vi "AprilTagFieldLayout_GetField.vi"(11 "AprilTagFieldLayout":T6={"AprilTagMap"={}, "FieldLength"=0.0, "FieldWidth"=0.0, "OriginPosition "=enum."kBlueAllianceWallRightSide,", "OriginPose3d"={"Translation3d"={"X"=0.0, "Y"=0.0, "Z"=0.0}, "Rotation3d"={"Q_quaternion"={"R"=1.0, "V"=[0.0, 0.0, 0.0]}}}} {"OriginPose3d"."Translation3d"."Z" format="%14.3f"; "OriginPose3d"."Translation3d"."Y" format="%14.3f"; "OriginPose3d"."Translation3d"."X" format="%14.3f"}) -> (0 "OriginPose3d":T1={"Translation3d"={"X"=0.0, "Y"=0.0, "Z"=0.0}, "Rotation3d"={"Q_quaternion"={"R"=1.0, "V"=[0.0, 0.0, 0.0]}}} {"Translation3d"."Z" format="%14.3f"; "Translation3d"."Y" format="%14.3f"; "Translation3d"."X" format="%14.3f"}, 1 "OriginPosition":T5, 2 "FieldWidth":dbl, 3 "FieldLength":dbl)   [LabVIEW 2019, in "Trajectory_Library.lvlib"]
doc: "Returns data about an AprilTagFieldLayout.\n\nInputs:\n -- AprilTagFIeldLayout -- AprilTagFieldLayout -- Data cluster \n\nOutputs:\n -- FieldLength -- double -- Field length (meters)\n -- FieldWidth -- double -- Field width (meters)\n -- OrginPosition -- enum -- Location of field origin\n -- OrignPose3d -- Pose3 -- Position of the field origin."
uses:
  Trajectory_Library.lvlib
  TypeDef/AprilTagFieldLayout.ctl
  TypeDef/AprilTag.ctl
  TypeDef/POSE3D.ctl
  TypeDef/TRANSLATION3D.ctl
  TypeDef/ROTATION3D.ctl
  TypeDef/QUATERNION.ctl
  Enum/AprilTagFieldLayoutOrignPosition_ENUM.ctl
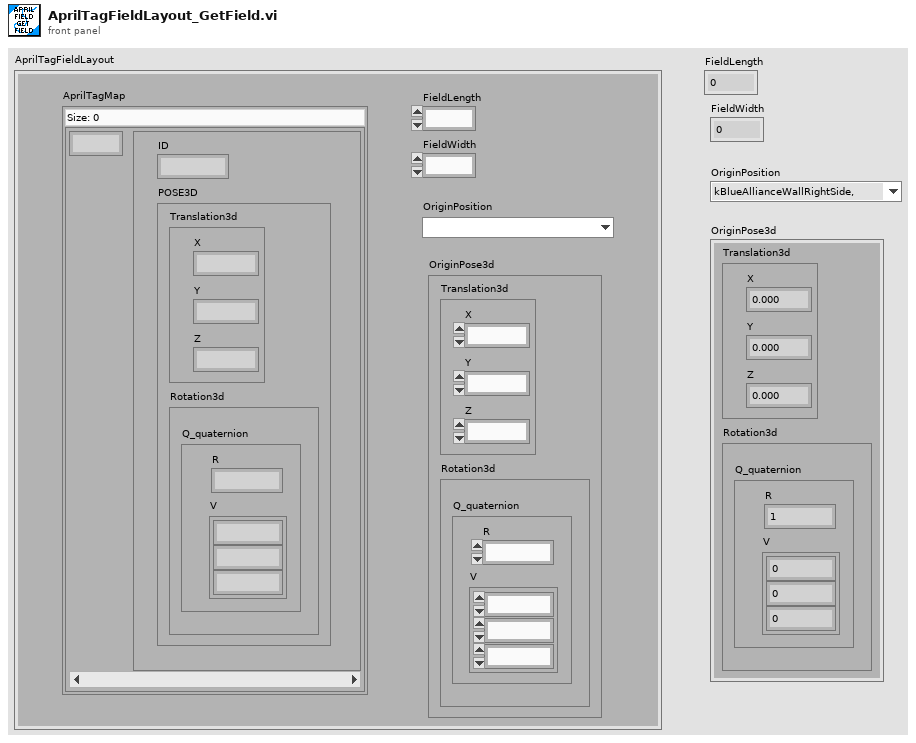
[diagram p1: front panel]
types:
  T1 = typedef "Trajectory_Library.lvlib/POSE3D.ctl" = cluster{"Translation3d":T2, "Rotation3d":T3}
  T2 = typedef "Trajectory_Library.lvlib/TRANSLATION3D.ctl" = cluster{"X":dbl, "Y":dbl, "Z":dbl}
  T3 = typedef "Trajectory_Library.lvlib/ROTATION3D.ctl" = cluster{"Q_quaternion":T4}
  T4 = typedef "Trajectory_Library.lvlib/QUATERNION.ctl" = cluster{"R":dbl, "V":dbl[]}
  T5 = typedef "Trajectory_Library.lvlib/AprilTagFieldLayoutOrignPosition_ENUM.ctl" = enum16{"kBlueAllianceWallRightSide,", "kRedAllianceWallRightSide,"}
  T6 = typedef "Trajectory_Library.lvlib/AprilTagFieldLayout.ctl" = cluster{"AprilTagMap":map{i32, T7}, "FieldLength":dbl, "FieldWidth":dbl, "OriginPosition ":T5, "OriginPose3d":T1}
  T7 = typedef "Trajectory_Library.lvlib/AprilTag.ctl" = cluster{"ID":i32, "POSE3D":T1}
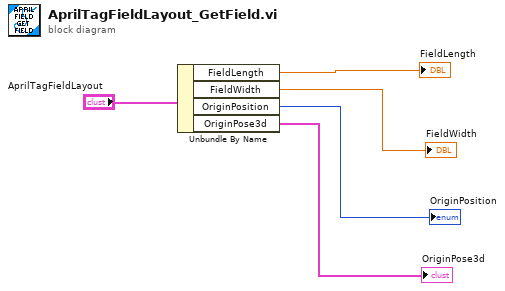
[diagram p0: block diagram]
diagram:
  n1 = Unbundle By Name("AprilTagFieldLayout") -> ("FieldLength"=→"FieldLength":dbl, "FieldWidth"=→"FieldWidth":dbl, "OriginPosition"=→"OriginPosition":T5, "OriginPose3d"=→"OriginPose3d":T1)
